vi "michsol.vi"(1 "LEFTOTRETE":bool) -> (0 "Boolean":bool)   [LabVIEW 2013]
uses:
  <vilib>/NXT/Block Support/NXT_OutputPort.ctl
  <vilib>/NXT/Block Support/NXT_InputPort.ctl
  <vilib>/NXT/NXTIO Xnodes/NXTIONodeSubVIs/NXTMoveMotors.vi
  <vilib>/NXT/Dual Mode Library/Sensors/EV3_Gyro_Angle.vi
  <vilib>/NXT/Dual Mode Library/Sensors/EV3_Ultrasonic_CM.vi
  <vilib>/NXT/Subs/LVHSConnector.ctl
  <vilib>/NXT/NXTIO Xnodes/AddressXNode/NXTIOAddress.xnode
  <vilib>/NXT/NXTIO Xnodes/NXTIOXNode/NXTIO.xnode
  <vilib>/NXT/LegoClasses/BrickReference/BrickReference.lvclass
panel:
  out "isWhite":bool
  out "isBlack":bool
  out "rightB":dbl
  out "leftA":dbl
  out "x > y?":bool
  out "Degrees":sgl
  out "x <= y?":bool
  in  "Numeric":dbl
  out "Centimeters":sgl
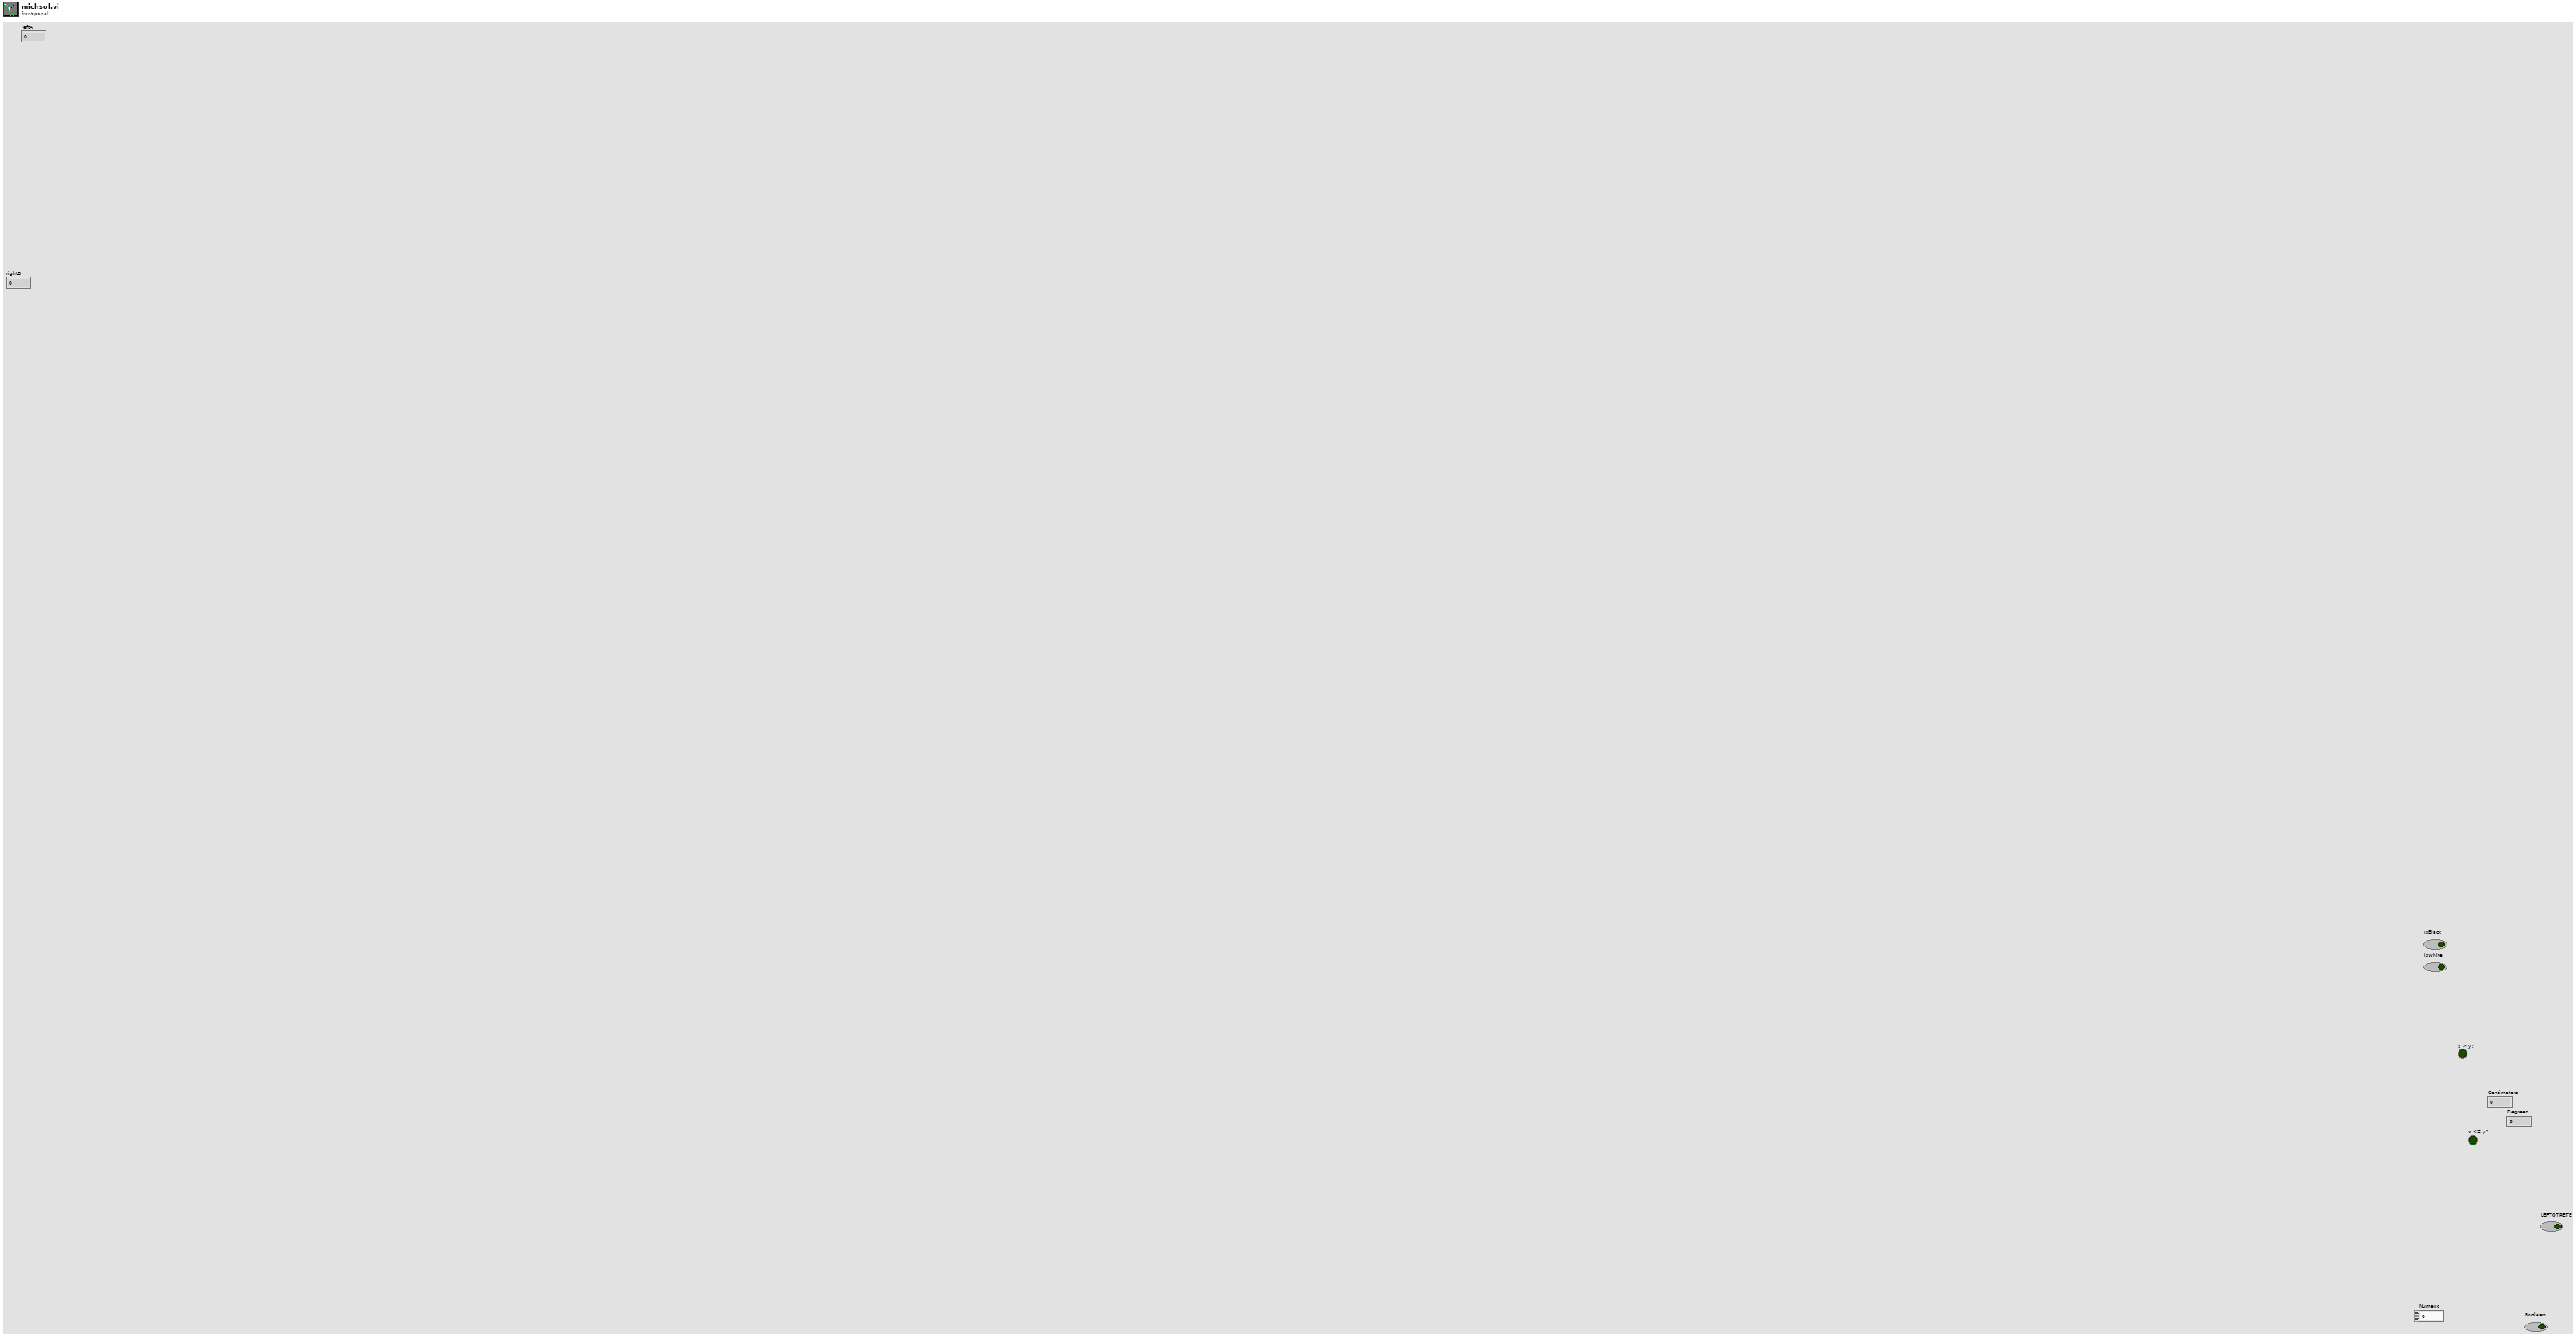
[diagram p1: front panel]
types:
  T1 = typedef "NXT_OutputPort.ctl" = u8
  T2 = typedef "NXT_InputPort.ctl" = u32
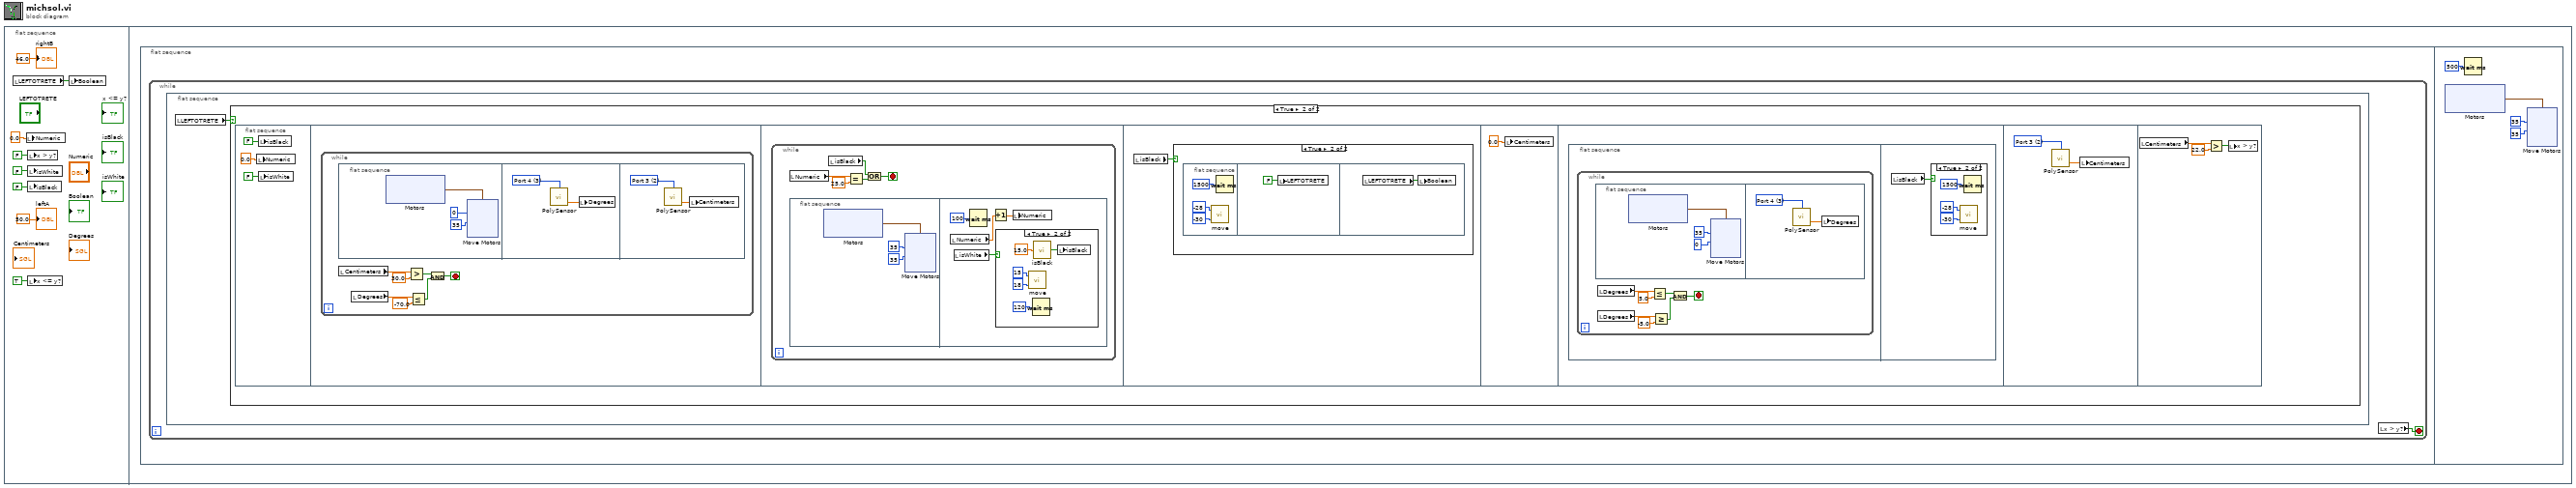
[diagram p0: block diagram]
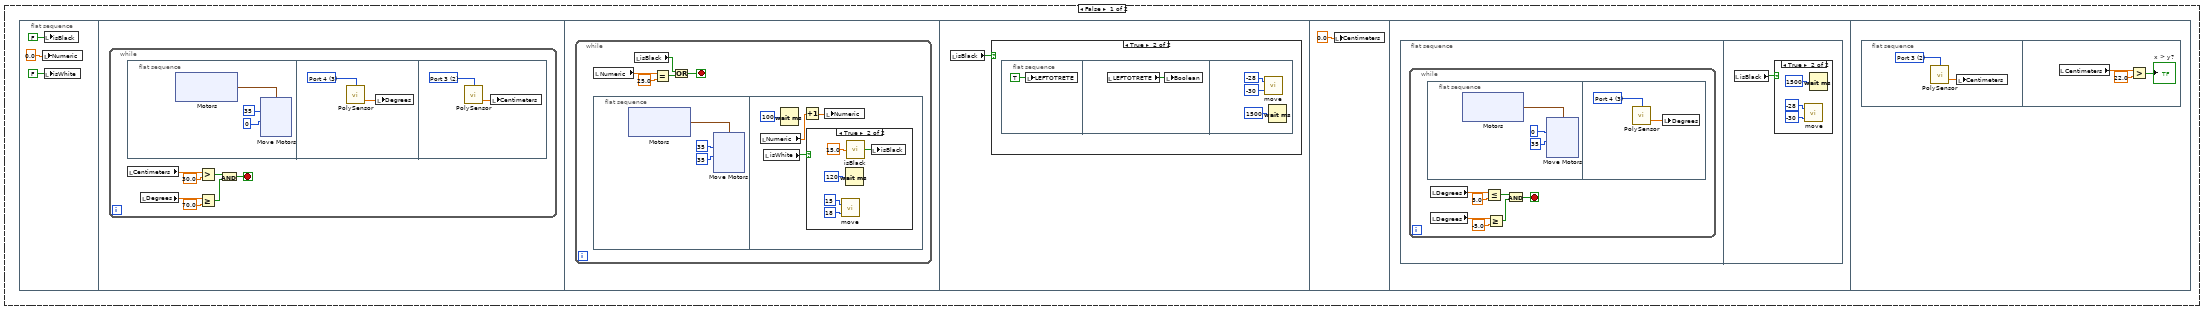
[diagram p2: hidden frame]
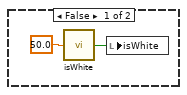
[diagram p3: hidden frame]
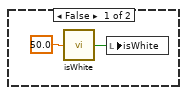
[diagram p6: hidden frame]
diagram:
  n1 = flat-sequence {
    frame #0 {
      n2 = local read "LEFTOTRETE"() -> (w1:bool)
      n3 = local write "Numeric"(0.0 ("Numeric")) -> ()
      n4 = local write "x > y?"(FALSE ("x > y?")) -> ()
      n5 = local write "isWhite"(FALSE ("isWhite")) -> ()
      n6 = local write "isBlack"(FALSE ("isBlack")) -> ()
      n7 = local write "x <= y?"(TRUE ("x <= y?")) -> ()
      n8 = local write "Boolean"(w1) -> ()
      "leftA" <- 50.0 ("leftA")
      "rightB" <- 46.0 ("Numeric")
    }
    frame #1 {
      n9 = flat-sequence {
        frame #0 {
          n10 = while {
            stop <- w9 stop-if-true
            n11 = flat-sequence {
              frame #0 {
                n12 = local read "LEFTOTRETE"() -> (w10:bool)
                n13 = case shown="True" w10 {
                  frame False {
                    n14 = flat-sequence {
                      frame #0 {
                        n15 = local write "Numeric"(0.0 ("Numeric")) -> ()
                        n16 = local write "isBlack"(FALSE ("isBlack")) -> ()
                        n17 = local write "isWhite"(FALSE ("isWhite")) -> ()
                      }
                      frame #1 {
                        n18 = while {
                          stop <- w14 stop-if-true
                          n19 = flat-sequence {
                            frame #0 {
                              n20 = xnode "Motors"() -> ("Motor"=w21:cluster{"Port":T1, "Port":T1})
                              n21 = xnode "Move Motors"("Power/Speed 2"=i8 0, "Power/Speed 1"=i8 35, "Motors"=w21) -> ()  [unwired: 1 in, 1 out]
                            }
                            frame #1 {
                              w34 = T2 3 items=["Port 1", "Port 2", "Port 3", "Port 4"] ("Port (Port 1)")
                              n22 = call-poly <vilib>:"PolySensor.vi"("Port (Port 1)"=w34) -> ("Degrees"=w33:sgl)  [unwired: 2 in, 1 out]
                              n23 = local write "Degrees"(w33) -> ()
                            }
                            frame #2 {
                              w36 = T2 2 items=["Port 1", "Port 2", "Port 3", "Port 4"] ("Port (Port 1)")
                              n24 = call-poly <vilib>:"PolySensor.vi"("Port (Port 1)"=w36) -> ("Centimeters"=w35:sgl)  [unwired: 2 in, 1 out]
                              n25 = local write "Centimeters"(w35) -> ()
                            }
                          }
                          n26 = local read "Centimeters"() -> (w18:sgl)
                          n27 = local read "Degrees"() -> (w20:sgl)
                          n28 = Greater?(x=w18, y=sgl 30.0) -> (0:w15:bool)
                          n29 = Greater Or Equal?(x=w20, y=sgl 70.0) -> (x >= y?=w16:bool)
                          n30 = And(x=w15, y=w16) -> (x .and. y?=w14:bool)
                        }
                      }
                      frame #2 {
                        n31 = while {
                          stop <- w37 stop-if-true
                          n32 = local read "Numeric"() -> (w40:dbl)
                          n33 = flat-sequence {
                            frame #0 {
                              n34 = xnode "Motors"() -> ("Motor"=w43:cluster{"Port":T1, "Port":T1})
                              n35 = xnode "Move Motors"("Power/Speed 2"=i8 35, "Power/Speed 1"=i8 35, "Motors"=w43) -> ()  [unwired: 1 in, 1 out]
                            }
                            frame #1 {
                              n36 = local read "Numeric"() -> (w57:dbl)
                              n37 = local read "isWhite"() -> (w54:bool)
                              n38 = Wait (ms)(milliseconds to wait=u32 100) -> ()  [unwired: 1 out]
                              n39 = Increment(x=w57) -> (x+1=w56:dbl)
                              n40 = case shown="True" w54 {
                                frame False {
                                n41 = call "isWhite.vi"("whiteBOND"=50.0) -> ("isWhite"=w58:bool)
                                n42 = local write "isWhite"(w58) -> ()
                                }
                                frame True {
                                n43 = call "move.vi"("speedLeft"=i8 18, "speedRight"=i8 15) -> ()  [unwired: 1 in]
                                n44 = Wait (ms)(milliseconds to wait=u32 120) -> ()  [unwired: 1 out]
                                n45 = call "isBlack.vi"("BlackBOND"=15.0) -> ("isBlack"=w63:bool)
                                n46 = local write "isBlack"(w63) -> ()
                                }
                              }
                              n47 = local write "Numeric"(w56) -> ()
                            }
                          }
                          n48 = local read "isBlack"() -> (w41:bool)
                          n49 = Equal?(x=w40, y=25.0) -> (x = y?=w38:bool)
                          n50 = Or(x=w41, y=w38) -> (x .or. y?=w37:bool)
                        }
                      }
                      frame #3 {
                        n51 = local read "isBlack"() -> (w65:bool)
                        n52 = case shown="True" w65 {
                          frame False {
                          }
                          frame True {
                            n53 = flat-sequence {
                              frame #0 {
                                n54 = local write "LEFTOTRETE"(TRUE ("LEFTOTRETE")) -> ()
                              }
                              frame #1 {
                                n55 = local read "LEFTOTRETE"() -> (w67:bool)
                                n56 = local write "Boolean"(w67) -> ()
                              }
                              frame #2 {
                                n57 = call "move.vi"("speedLeft"=i8 -30, "speedRight"=i8 -28) -> ()  [unwired: 1 in]
                                n58 = Wait (ms)(milliseconds to wait=u32 1500) -> ()  [unwired: 1 out]
                              }
                            }
                          }
                        }
                      }
                      frame #4 {
                        n59 = local write "Centimeters"(sgl 0.0 ("Centimeters")) -> ()
                      }
                      frame #5 {
                        n60 = flat-sequence {
                          frame #0 {
                            n61 = while {
                              stop <- w72 stop-if-true
                              n62 = flat-sequence {
                                frame #0 {
                                n63 = xnode "Motors"() -> ("Motor"=w80:cluster{"Port":T1, "Port":T1})
                                n64 = xnode "Move Motors"("Power/Speed 2"=i8 35, "Power/Speed 1"=i8 0, "Motors"=w80) -> ()  [unwired: 1 in, 1 out]
                                }
                                frame #1 {
                                w92 = T2 3 items=["Port 1", "Port 2", "Port 3", "Port 4"] ("Port (Port 1)")
                                n65 = call-poly <vilib>:"PolySensor.vi"("Port (Port 1)"=w92) -> ("Degrees"=w91:sgl)  [unwired: 2 in, 1 out]
                                n66 = local write "Degrees"(w91) -> ()
                                }
                              }
                              n67 = local read "Degrees"() -> (w78:sgl)
                              n68 = local read "Degrees"() -> (w75:sgl)
                              n69 = Less Or Equal?(x=w78, y=sgl 5.0) -> (x <= y?=w73:bool)
                              n70 = Greater Or Equal?(x=w75, y=-5.0) -> (x >= y?=w74:bool)
                              n71 = And(x=w73, y=w74) -> (x .and. y?=w72:bool)
                            }
                          }
                          frame #1 {
                            n72 = local read "isBlack"() -> (w93:bool)
                            n73 = case shown="True" w93 {
                              frame False {
                              }
                              frame True {
                                n74 = call "move.vi"("speedLeft"=i8 -30, "speedRight"=i8 -28) -> ()  [unwired: 1 in]
                                n75 = Wait (ms)(milliseconds to wait=u32 1500) -> ()  [unwired: 1 out]
                              }
                            }
                          }
                        }
                      }
                      frame #6 {
                        n76 = flat-sequence {
                          frame #0 {
                            w97 = T2 2 items=["Port 1", "Port 2", "Port 3", "Port 4"] ("Port (Port 1)")
                            n77 = call-poly <vilib>:"PolySensor.vi"("Port (Port 1)"=w97) -> ("Centimeters"=w98:sgl)  [unwired: 2 in, 1 out]
                            n78 = local write "Centimeters"(w98) -> ()
                          }
                          frame #1 {
                            n79 = local read "Centimeters"() -> (w100:sgl)
                            n80 = Greater?(x=w100, y=sgl 22.0) -> (0:→"x > y?":bool)
                          }
                        }
                      }
                    }
                  }
                  frame True {
                    n81 = flat-sequence {
                      frame #0 {
                        n82 = local write "Numeric"(0.0 ("Numeric")) -> ()
                        n83 = local write "isBlack"(FALSE ("isBlack")) -> ()
                        n84 = local write "isWhite"(FALSE ("isWhite")) -> ()
                      }
                      frame #1 {
                        n85 = while {
                          stop <- w105 stop-if-true
                          n86 = flat-sequence {
                            frame #0 {
                              n87 = xnode "Motors"() -> ("Motor"=w113:cluster{"Port":T1, "Port":T1})
                              n88 = xnode "Move Motors"("Power/Speed 2"=i8 35, "Power/Speed 1"=i8 0, "Motors"=w113) -> ()  [unwired: 1 in, 1 out]
                            }
                            frame #1 {
                              w124 = T2 3 items=["Port 1", "Port 2", "Port 3", "Port 4"] ("Port (Port 1)")
                              n89 = call-poly <vilib>:"PolySensor.vi"("Port (Port 1)"=w124) -> ("Degrees"=w125:sgl)  [unwired: 2 in, 1 out]
                              n90 = local write "Degrees"(w125) -> ()
                            }
                            frame #2 {
                              w127 = T2 2 items=["Port 1", "Port 2", "Port 3", "Port 4"] ("Port (Port 1)")
                              n91 = call-poly <vilib>:"PolySensor.vi"("Port (Port 1)"=w127) -> ("Centimeters"=w126:sgl)  [unwired: 2 in, 1 out]
                              n92 = local write "Centimeters"(w126) -> ()
                            }
                          }
                          n93 = local read "Centimeters"() -> (w109:sgl)
                          n94 = local read "Degrees"() -> (w111:sgl)
                          n95 = Greater?(x=w109, y=sgl 30.0) -> (0:w107:bool)
                          n96 = Less Or Equal?(x=w111, y=-70.0) -> (x <= y?=w106:bool)
                          n97 = And(x=w107, y=w106) -> (x .and. y?=w105:bool)
                        }
                      }
                      frame #2 {
                        n98 = while {
                          stop <- w128 stop-if-true
                          n99 = local read "Numeric"() -> (w131:dbl)
                          n100 = flat-sequence {
                            frame #0 {
                              n101 = xnode "Motors"() -> ("Motor"=w134:cluster{"Port":T1, "Port":T1})
                              n102 = xnode "Move Motors"("Power/Speed 2"=i8 35, "Power/Speed 1"=i8 35, "Motors"=w134) -> ()  [unwired: 1 in, 1 out]
                            }
                            frame #1 {
                              n103 = local read "Numeric"() -> (w148:dbl)
                              n104 = local read "isWhite"() -> (w145:bool)
                              n105 = Wait (ms)(milliseconds to wait=u32 100) -> ()  [unwired: 1 out]
                              n106 = Increment(x=w148) -> (x+1=w147:dbl)
                              n107 = case shown="True" w145 {
                                frame False {
                                n108 = call "isWhite.vi"("whiteBOND"=50.0) -> ("isWhite"=w150:bool)
                                n109 = local write "isWhite"(w150) -> ()
                                }
                                frame True {
                                n110 = call "move.vi"("speedLeft"=i8 18, "speedRight"=i8 15) -> ()  [unwired: 1 in]
                                n111 = Wait (ms)(milliseconds to wait=u32 120) -> ()  [unwired: 1 out]
                                n112 = call "isBlack.vi"("BlackBOND"=15.0) -> ("isBlack"=w154:bool)
                                n113 = local write "isBlack"(w154) -> ()
                                }
                              }
                              n114 = local write "Numeric"(w147) -> ()
                            }
                          }
                          n115 = local read "isBlack"() -> (w132:bool)
                          n116 = Equal?(x=w131, y=25.0) -> (x = y?=w129:bool)
                          n117 = Or(x=w132, y=w129) -> (x .or. y?=w128:bool)
                        }
                      }
                      frame #3 {
                        n118 = local read "isBlack"() -> (w156:bool)
                        n119 = case shown="True" w156 {
                          frame False {
                          }
                          frame True {
                            n120 = flat-sequence {
                              frame #0 {
                                n121 = call "move.vi"("speedLeft"=i8 -30, "speedRight"=i8 -28) -> ()  [unwired: 1 in]
                                n122 = Wait (ms)(milliseconds to wait=u32 1500) -> ()  [unwired: 1 out]
                              }
                              frame #1 {
                                n123 = local write "LEFTOTRETE"(FALSE ("LEFTOTRETE")) -> ()
                              }
                              frame #2 {
                                n124 = local read "LEFTOTRETE"() -> (w161:bool)
                                n125 = local write "Boolean"(w161) -> ()
                              }
                            }
                          }
                        }
                      }
                      frame #4 {
                        n126 = local write "Centimeters"(sgl 0.0 ("Centimeters")) -> ()
                      }
                      frame #5 {
                        n127 = flat-sequence {
                          frame #0 {
                            n128 = while {
                              stop <- w163 stop-if-true
                              n129 = flat-sequence {
                                frame #0 {
                                n130 = xnode "Motors"() -> ("Motor"=w171:cluster{"Port":T1, "Port":T1})
                                n131 = xnode "Move Motors"("Power/Speed 2"=i8 0, "Power/Speed 1"=i8 35, "Motors"=w171) -> ()  [unwired: 1 in, 1 out]
                                }
                                frame #1 {
                                w183 = T2 3 items=["Port 1", "Port 2", "Port 3", "Port 4"] ("Port (Port 1)")
                                n132 = call-poly <vilib>:"PolySensor.vi"("Port (Port 1)"=w183) -> ("Degrees"=w182:sgl)  [unwired: 2 in, 1 out]
                                n133 = local write "Degrees"(w182) -> ()
                                }
                              }
                              n134 = local read "Degrees"() -> (w169:sgl)
                              n135 = local read "Degrees"() -> (w166:sgl)
                              n136 = Less Or Equal?(x=w169, y=sgl 5.0) -> (x <= y?=w164:bool)
                              n137 = Greater Or Equal?(x=w166, y=-5.0) -> (x >= y?=w165:bool)
                              n138 = And(x=w164, y=w165) -> (x .and. y?=w163:bool)
                            }
                          }
                          frame #1 {
                            n139 = local read "isBlack"() -> (w184:bool)
                            n140 = case shown="True" w184 {
                              frame False {
                              }
                              frame True {
                                n141 = call "move.vi"("speedLeft"=i8 -30, "speedRight"=i8 -28) -> ()  [unwired: 1 in]
                                n142 = Wait (ms)(milliseconds to wait=u32 1500) -> ()  [unwired: 1 out]
                              }
                            }
                          }
                        }
                      }
                      frame #6 {
                        w189 = T2 2 items=["Port 1", "Port 2", "Port 3", "Port 4"] ("Port (Port 1)")
                        n143 = call-poly <vilib>:"PolySensor.vi"("Port (Port 1)"=w189) -> ("Centimeters"=w188:sgl)  [unwired: 2 in, 1 out]
                        n144 = local write "Centimeters"(w188) -> ()
                      }
                      frame #7 {
                        n145 = local read "Centimeters"() -> (w192:sgl)
                        n146 = Greater?(x=w192, y=sgl 22.0) -> (0:w190:bool)
                        n147 = local write "x > y?"(w190) -> ()
                      }
                    }
                  }
                }
              }
            }
            n148 = local read "x > y?"() -> (w9:bool)
          }
        }
        frame #1 {
          n149 = xnode "Motors"() -> ("Motor"=w195:cluster{"Port":T1, "Port":T1})
          n150 = Wait (ms)(milliseconds to wait=u32 500) -> ()  [unwired: 1 out]
          n151 = xnode "Move Motors"("Power/Speed 2"=i8 35, "Power/Speed 1"=i8 35, "Motors"=w195) -> ()  [unwired: 1 in, 1 out]
        }
      }
    }
  }
